vi "UT - Create and Write to HDF File.vi"(8 "error in (no error)":errorcluster, 10 "indices":u64[](array[numeric]), 11 "Dims":u64[](array[numeric])) -> (0 "error out":errorcluster, 3 "data":dbl)   [LabVIEW 2019]
uses:
  <vilib>/UPVI/lvhdf5/file.llb/LVH5F Operation.ctl
  <vilib>/UPVI/lvhdf5/group.llb/H5G_obj_t.ctl
  <vilib>/Utility/miscctls.llb/LVRectTypeDef.ctl
  <vilib>/UPVI/lvhdf5/dataset.llb/LVH5D Operation.ctl
  <vilib>/UPVI/lvhdf5/utility.llb/Select HDF5 Dialog.vi
  <vilib>/UPVI/lvhdf5/utility.llb/Select HDF5 Dialog (Object Only).vi
  <vilib>/UPVI/lvhdf5/dataset.llb/Simple H5Dread (Variant).vi
  <vilib>/UPVI/lvhdf5/dataset.llb/Simple H5Dread.xnode
  <vilib>/UPVI/lvhdf5/library.llb/HDF5 Ref.ctl
  HDF5 Tools.lvlib
  <vilib>/UPVI/lvhdf5/file.llb/H5Fopen.vi
  <vilib>/UPVI/lvhdf5/identifier.llb/Not an HDF5 Refnum Constant.vi
  <vilib>/UPVI/lvhdf5/dataset.llb/OpenCreateReplace Dataset.vi
  <vilib>/UPVI/lvhdf5/dataset.llb/H5Dget_space.vi
  <vilib>/UPVI/lvhdf5/dataspace.llb/H5Sget_simple_extent_dims.vi
  <vilib>/UPVI/lvhdf5/dataspace.llb/H5Sselect_hyperslab.vi
  <vilib>/UPVI/lvhdf5/dataset.llb/H5Dread (Variant).vi
  <vilib>/UPVI/lvhdf5/attribute.llb/private/LVH5AreadWDTAttrs.vi
  <vilib>/UPVI/lvhdf5/dataspace.llb/H5Sclose.vi
  <vilib>/Utility/error.llb/Error Cluster From Error Code.vi
  <vilib>/UPVI/lvhdf5/dataset.llb/H5Dclose.vi
  <vilib>/UPVI/lvhdf5/utility.llb/Select HDF5 Dialog (File and Object).vi
panel:
  out "Object Names":string[](array[string])
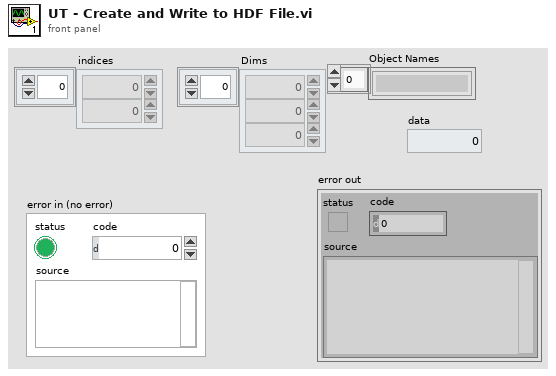
[diagram p1: front panel]
types:
  T1 = typedef "LVH5F Operation.ctl" = enum16{"open", "open or create", "create or replace", "create or replace (with confirmation)", "create", "open (read only)"}
  T2 = typedef "LVRectTypeDef.ctl" = cluster{"Left":i16, "Top":i16, "Right":i16, "Bottom":i16}
  T3 = cluster{"Behavior":enum32{"Invalid", "Default", "Floating", "Floating/Auto-Hide", "Modal"}, "Position":T2, "Center":bool, "Title":string}
  T4 = typedef "LVH5D Operation.ctl" = enum16{"open", "replace", "create", "open or create", "create or replace", "create or replace with confirmation"}
  T5 = typedef "H5G_obj_t.ctl" = i32
  T6 = cluster{"Object Types (any)":T5[], "Object Pattern":string}
  T7 = cluster{"My Numeric":dbl, "My Array":dbl[][], "My Inner Cluster":cluster{"My Numeric in Cluster":dbl}}
  T8 = typedef "HDF5 Ref.ctl" = refnum<k1>
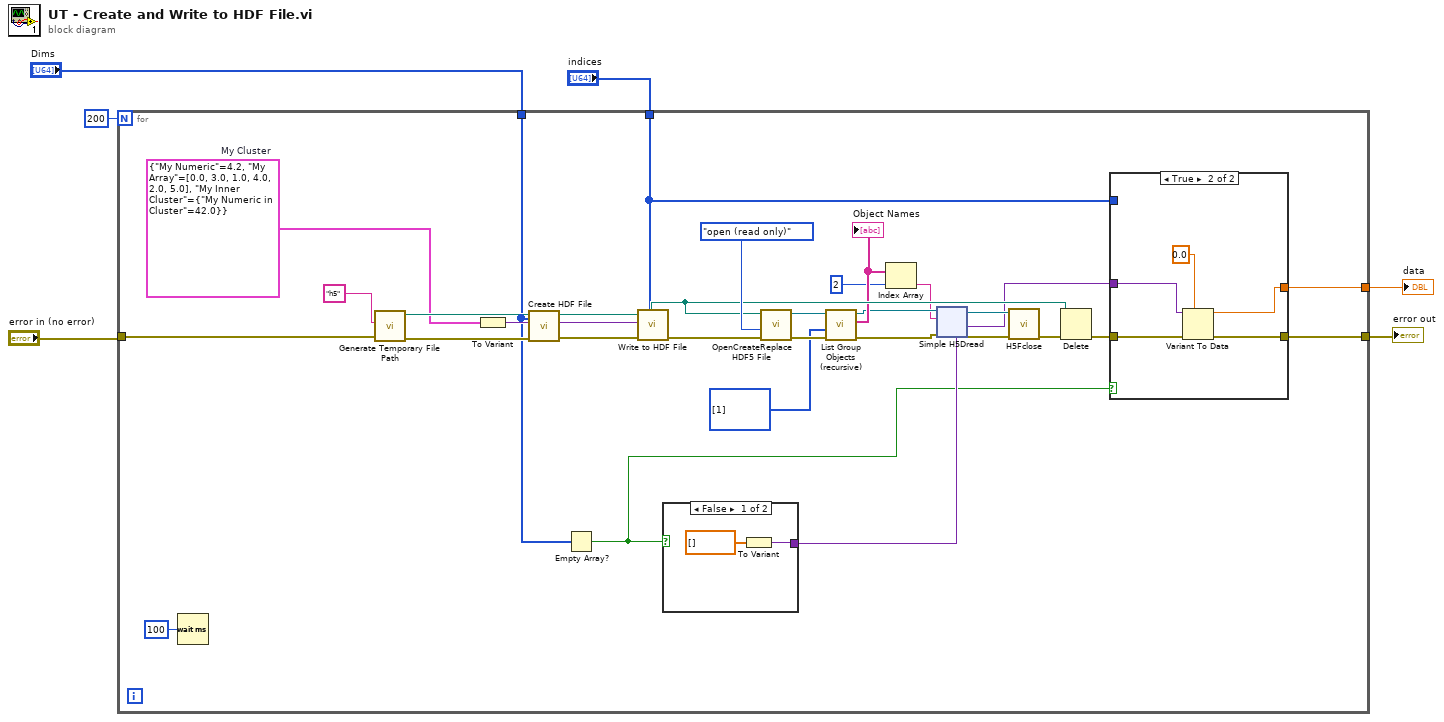
[diagram p0: block diagram]
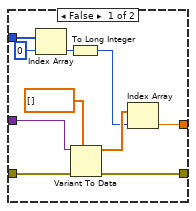
[diagram p2: hidden frame]
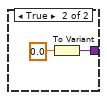
[diagram p3: hidden frame]
diagram:
  n1 = for {
    N: 200 -> [_]
    tunnel: "Dims" -> [w24]
    tunnel: "indices" -> [w9]
    tunnel: [w8] -> w2
    tunnel: "error in (no error)" -> [w34]
    tunnel: [w11] -> w4
    w17 = T5[] [1] items=["H5G_UNKNOWN"=-1, "H5G_GROUP"=0, "H5G_DATASET"=1, "H5G_TYPE"=2, "H5G_LINK"=3, "H5G_UDLINK"=4] ("Object Types (any)")
    w30 = T7 {"My Numeric"=4.2, "My Array"=[[0.0, 3.0], [1.0, 4.0], [2.0, 5.0]], "My Inner Cluster"={"My Numeric in Cluster"=42.0}}  # My Cluster
    n2 = Wait (ms)(milliseconds to wait=u32 100) -> ()  [unwired: 1 out]
    n3 = call <vilib>:"Generate Temporary File Path.vi"("error in (no error)"=w34, "Temporary File Extension (tmp)"="h5") -> ("error out"=w35:errorcluster, "Unique Temporary File Path"=w33:path)  [unwired: 8 in]
    n4 = To Variant(anything=w30) -> (Variant=w31:variant)
    n5 = call "Create HDF File.vi"("Dims"=w24, "error in (no error)"=w35, "variant"=w31, "path"=w33) -> ("error out"=w37:errorcluster, "variant out"=w26:variant, "path out"=w25:path)  [unwired: 5 in]
    n6 = Empty Array?(array=w24) -> (empty?=w13:bool)
    n7 = call "Write to HDF File.vi"("indices"=w9, "error in (no error)"=w37, "variant"=w26, "path"=w25) -> ("error out"=w23:errorcluster)  [unwired: 7 in]
    n8 = case shown="False" w13 {
      tunnel: [w53 w55] -> w14
      frame False {
        n9 = To Variant(anything=dbl[] []) -> (Variant=w53:variant)
      }
      frame True {
        n10 = To Variant(anything=0.0) -> (Variant=w55:variant)
      }
    }
    n11 = call <vilib>:"OpenCreateReplace HDF5 File.vi"("error in (no error)"=w23, "function (open or create)"=LVH5F_Operation."open (read only)", "path"=w25) -> ("error out"=w20:errorcluster, "HDF5 Ref out"=w22:T8)  [unwired: 5 in]
    n12 = call <vilib>:"List Group Objects (recursive).vi"("error in (no error)"=w20, "Object Types (any)"=w17, "HDF5 Loc Ref"=w22) -> ("error out"=w19:errorcluster, "Object Names"=w21:string[], "HDF5 Loc Ref out"=w18:T8)  [unwired: 3 in, 1 out]
    "Object Names" <- w21
    n13 = Index Array(array=w21, index=2) -> (element=w16:string)
    n14 = xnode "Simple H5Dread"("Dataset Path"=w16, "error in (no error)"=w19, "HDF5 Path or Ref"=w18, "Data"=w14) -> ("HDF5 Ref out"=w29:T8, "error out"=w28:errorcluster, "Data out"=w10:variant)  [unwired: 1 out]
    n15 = call <vilib>:"H5Fclose.vi"("error in (no error)"=w28, "HDF5 Ref"=w29) -> ("error out"=w27:errorcluster)  [unwired: 7 in]
    n16 = Delete(path (use dialog)=w25, error in=w27) -> (error out=w12:errorcluster)  [unwired: 3 in, 2 out]
    n17 = case shown="True" w13 {
      tunnel: w12 -> [w47 w52]
      tunnel: [w46 w51] -> w11
      tunnel: w10 -> [w45 w50]
      tunnel: w9 -> [w43 _]
      tunnel: [w38 w48] -> w8
      frame False {
        n18 = Index Array(array=w43, index=0) -> (element=w40:u64)
        n19 = To Long Integer(number=w40) -> (32bit integer=w39:i32)
        n20 = Variant To Data(error in=w47, type=dbl[] [], Variant=w45) -> (data=w41:dbl[], error out=w46:errorcluster)
        n21 = Index Array(array=w41, index=w39) -> (element=w38:dbl)
      }
      frame True {
        n22 = Variant To Data(error in=w52, type=0.0, Variant=w50) -> (data=w48:dbl, error out=w51:errorcluster)
      }
    }
  }
  "error out" <- w4
  "data" <- w2
